vi "test_Read I8 Register Value.vi"(8 "error in (no error)":errorcluster, 11 "TestCase in":refnum<class "FPGA Register IO Tests.lvclass">=refnum) -> (0 "error out":errorcluster, 3 "TestCase out":refnum<class "FPGA Register IO Tests.lvclass">)   [LabVIEW 2026, in "FPGA Register IO Tests.lvclass"]
uses:
  FPGA Register IO Tests.lvclass
  FPGA Register IO Tests.lvclass/FPGA Register IO Tests.ctl
  APIs/FPGA Register IO/FPGA Register IO.lvlib
  FPGA Addon Test Class/FPGA Addon Test Class.lvclass
  Addon/Addon Engine/FPGA Addon Engine.lvlib
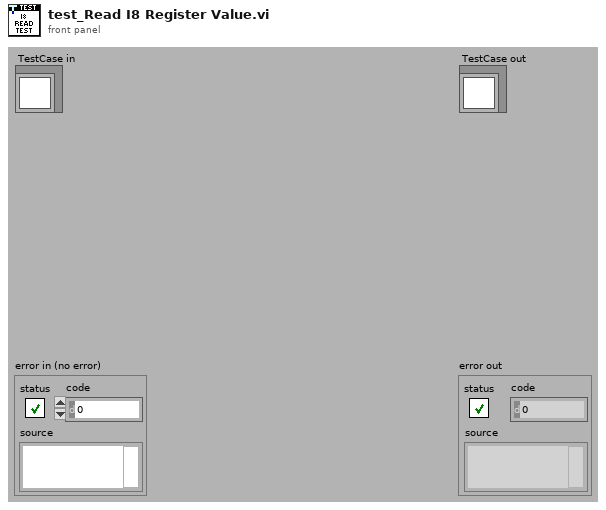
[diagram p1: front panel]
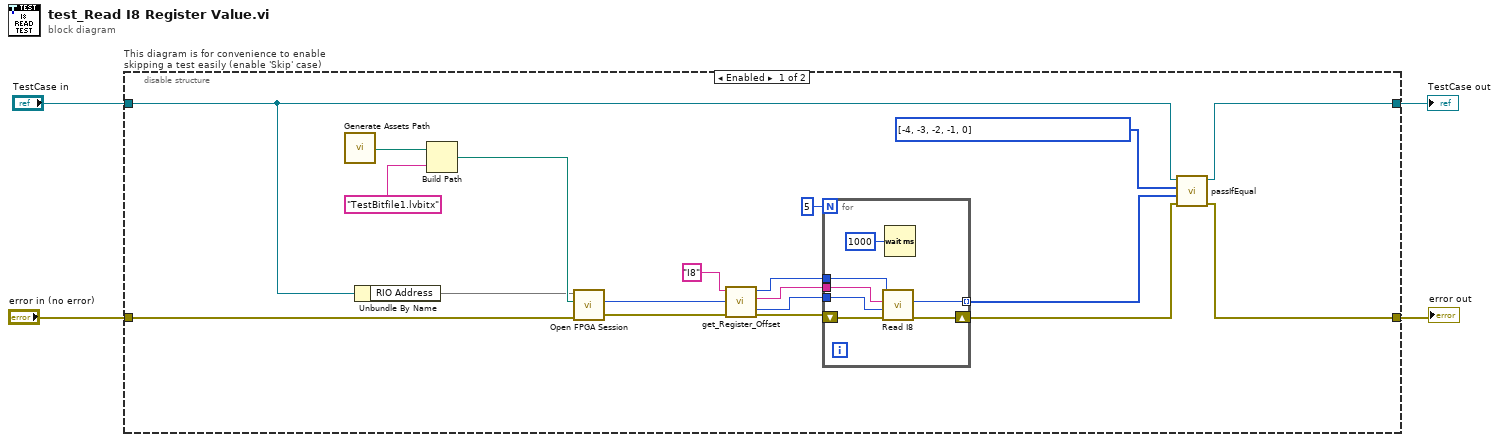
[diagram p0: block diagram]
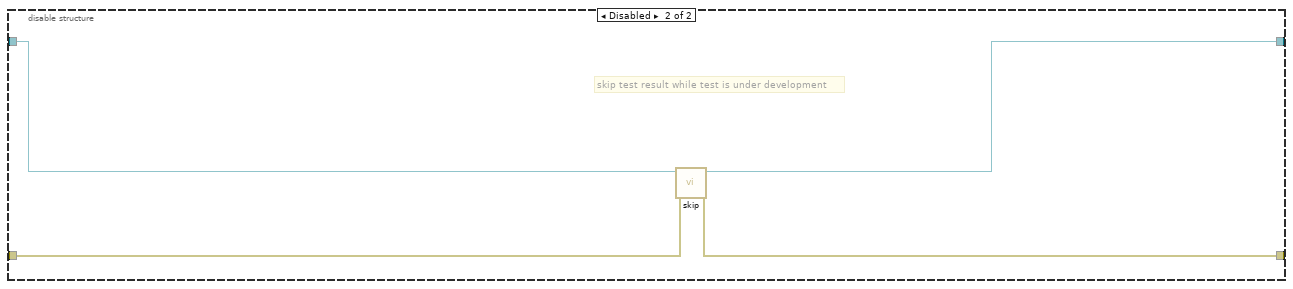
[diagram p2: hidden frame]
diagram:
  n1 = disable-structure "This diagram is for convenience to enable skipping a test easily (enable 'Skip' case)" shown="Enabled" {
    disable-tunnel: "TestCase in" -> [w16 w34]
    disable-tunnel: [w15 w32] -> w1
    disable-tunnel: [w14 w33] -> w3
    disable-tunnel: "error in (no error)" -> [w22 w31]
    frame Enabled {
      n2 = call "Generate Assets Path.vi"() -> ("Assets path"=w20:path)
      n3 = Unbundle By Name(w16) -> ("RIO Address"=w18)
      n4 = Build Path(base path=w20, name or relative path="TestBitfile1.lvbitx") -> (appended path=w19:path)
      n5 = call "Open FPGA Session.vi"("error in"=w22, "bitfile path"=w19, "device address"=w18) -> ("error out"=w9:errorcluster, "session out"=w10:u32)  [unwired: 6 in, 1 out]
      n6 = call "get_Register_Offset.vi"("error in (no error)"=w9, "session"=w10, "Name"="I8" ("register name")) -> ("error out"=w8:errorcluster, "RegisterOffset"=w5:u32, "Register Name"=w6:string, "session out"=w7:u32)  [unwired: 5 in]
      n7 = for {
        N: 5 -> [_]
        shift-right: [w29] -> w13
        shift-left: w8 -> [w30]
        tunnel: [w28] -> w12 mode=indexing
        tunnel: w7 -> [w26]
        tunnel: w6 -> [w25]
        tunnel: w5 -> [w24]
        n8 = call "Read I8.vi"("error in"=w30, "RegisterOffset"=w24, "register name"=w25, "session in"=w26) -> ("error out"=w29:errorcluster, "value out"=w28:i8)  [unwired: 5 in, 1 out]
        n9 = Wait (ms)(milliseconds to wait=u32 1000) -> ()  [unwired: 1 out]
      }
      n10 = call-dynamic "passIfEqual.vi"("error in (no error)"=w13, "y"=w12, "x"=i8[] [-4, -3, -2, -1, 0] ("Array"), "TestCase in"=w16) -> ("error out"=w14:errorcluster, "TestCase out"=w15:refnum<class "FPGA Register IO Tests.lvclass">)  [unwired: 6 in]
    }
    frame Disabled {
      # "skip test result while test is under development"
      n11 = call <vilib>:"skip.vi"("error in (no error)"=w31, "TestCase in"=w34) -> ("error out"=w33:errorcluster, "TestCase out"=w32:refnum<class "FPGA Register IO Tests.lvclass">)  [unwired: 8 in]
    }
  }
  "error out" <- w3
  "TestCase out" <- w1
